vi "Get Objects Available for PDO.vi"(8 "error in":errorcluster, 11 "Sorted Object Dictionary in":refnum<class "Sorted Object Dictionary.lvclass">) -> (0 "error out":errorcluster, 2 "Entries":refnum<class "OD Entry.lvclass">[](array[class]), 3 "Sorted Object Dictionary out":refnum<class "Sorted Object Dictionary.lvclass">)   [LabVIEW 2024, in "EDS.lvlib" / "Sorted Object Dictionary.lvclass"]
uses:
  Sorted Object Dictionary.lvclass
  Sorted Object Dictionary.lvclass/Sorted Object Dictionary.ctl
  OD Entry/OD Entry.lvclass
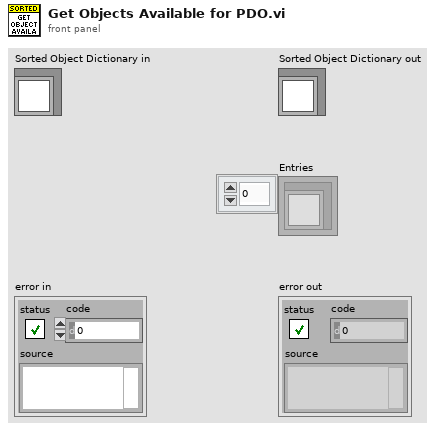
[diagram p1: front panel]
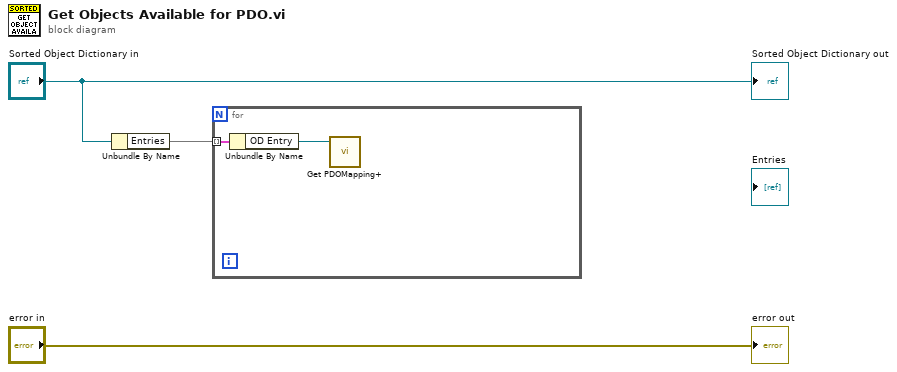
[diagram p0: block diagram]
diagram:
  n1 = Unbundle By Name("Sorted Object Dictionary in") -> ("Entries"=w1:map{u16, refnum<class "OD Entry.lvclass">})
  n2 = for {
    tunnel: w1 -> [w5] mode=indexing
    n3 = Unbundle By Name(w5) -> ("OD Entry"=w4:refnum<class "OD Entry.lvclass">)
    n4 = call "Get PDOMapping+.vi"("reference in"=w4) -> ()  [unwired: 7 in, 4 out]
  }
  "error out" <- "error in"
  "Sorted Object Dictionary out" <- "Sorted Object Dictionary in"
